vi "Termometros (1).vi"() -> ()   [LabVIEW 2025]
uses:
  control termometros.ctl
panel:
  out "Fahrenheit":dbl(knob) scale=32.0..300.0
  out "Kelvin":dbl(knob) scale=273.0..300.0
  out "Celsius":dbl(knob) scale=0.0..100.0
  out "Frio":bool
  out "Caliente":bool
  out "Kelvin":T1 scale=273.0..373.0
  out "Fahrenheit":dbl(slide) scale=32.0..300.0
  out "Celsius":dbl(slide) scale=0.0..100.0
  in  "Slide":dbl(slide) scale=0.0..100.0
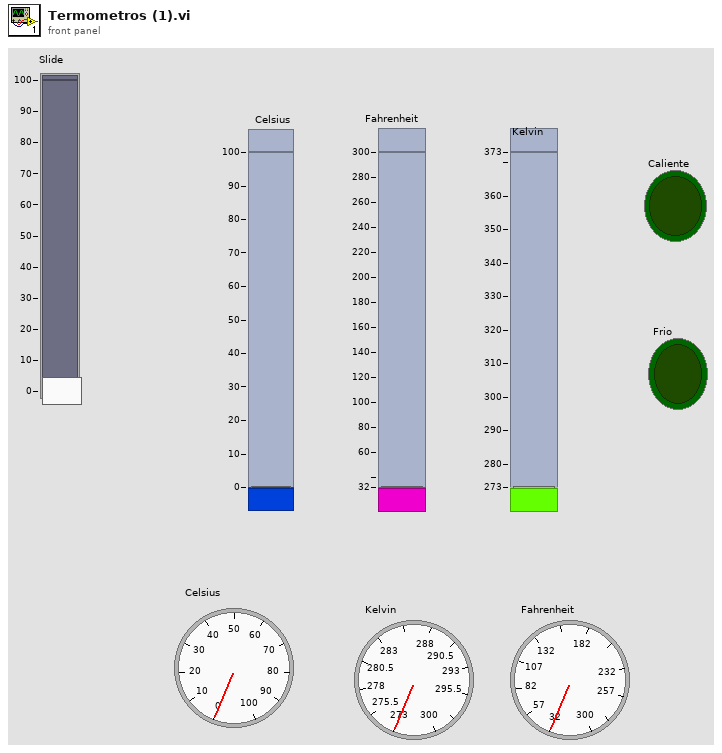
[diagram p1: front panel]
types:
  T1 = typedef "control termometros.ctl" = dbl
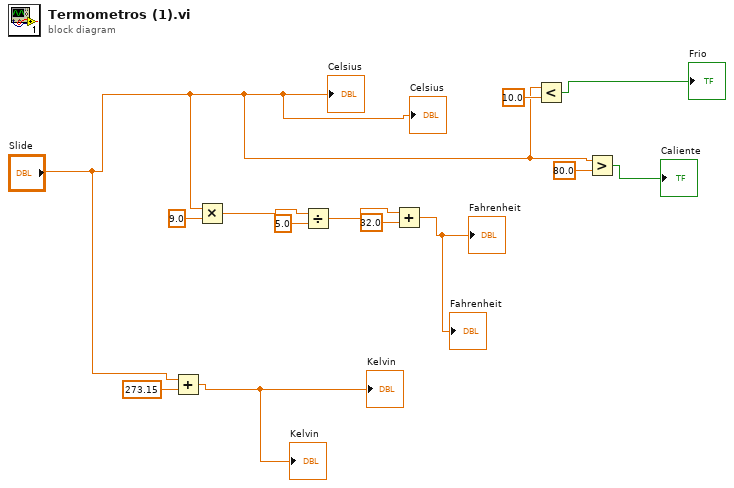
[diagram p0: block diagram]
diagram:
  n1 = Add(x="Slide", y=273.15) -> (x+y=→"Kelvin" →"Kelvin":dbl)
  n2 = Multiply(x="Slide", y=9.0) -> (x*y=w7:dbl)
  n3 = Divide(x=w7, y=5.0) -> (x/y=w6:dbl)
  n4 = Add(x=w6, y=32.0) -> (x+y=→"Fahrenheit" →"Fahrenheit":dbl)
  n5 = Less?(x="Slide", y=10.0) -> (x < y?=→"Frio":bool)
  n6 = Greater?(x="Slide", y=80.0) -> (0:→"Caliente":bool)
  "Celsius" <- "Slide"
  "Celsius" <- "Slide"
